vi "Evaluate Car Position.vi"(7 "Timeout":i32=-1, 11 "Car Wash Station Sequencer in":refnum<class "Car Wash Station Sequencer.lvclass">) -> (3 "Car Wash Station Sequencer out":refnum<class "Car Wash Station Sequencer.lvclass">, 5 "Timeout out":i32)   [LabVIEW 2016, in "CLD Exam - Car Wash.lvlib" / "Car Wash Station Sequencer.lvclass"]
uses:
  Car Wash Station Sequencer.lvclass
  D:/Repos/Stream/software/Mediator/Classes/Mediated Actor/Mediated Actor.lvclass
  Car Wash Station Sequencer.lvclass/Car Wash Station Sequencer.ctl
  Car Wash Finished Event/Car Wash Finished.lvclass
  D:/Repos/Stream/software/Mediator/Classes/Message Interface/Message Interface.lvclass
  Car Out of Position Event/Car Out of Position.lvclass
  Mediator/Classes/Message Interface/Message Interface.lvclass
  Car Wash Option Started Event/Car Wash Option Started.lvclass
  Mediator/Classes/Message Transport Queue/Message Transport Queue.lvclass
  Mediator/Classes/Mediated Actor/Mediated Actor.lvclass
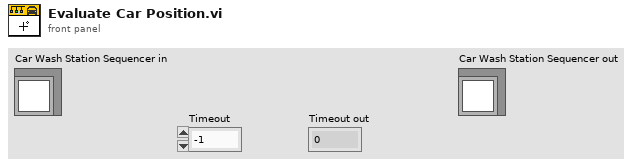
[diagram p1: front panel]
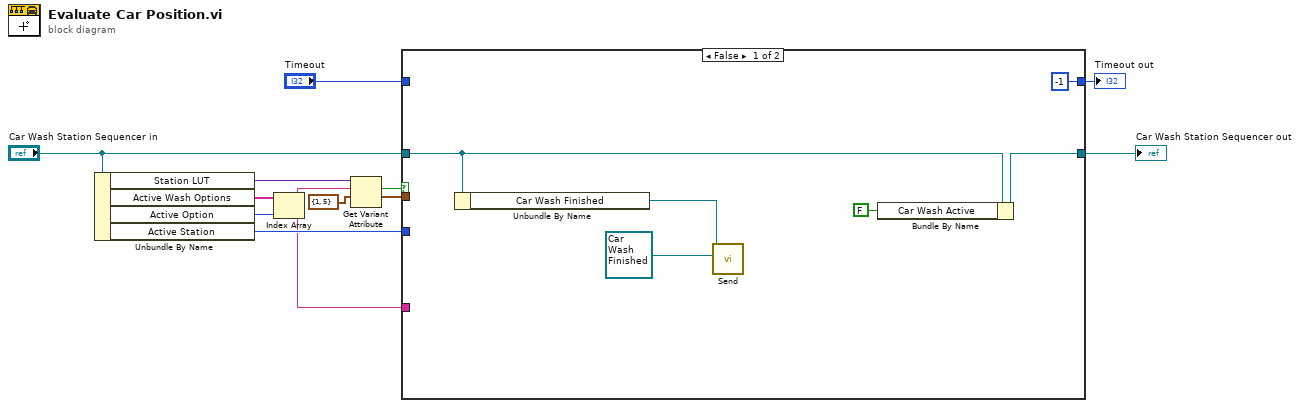
[diagram p0: block diagram]
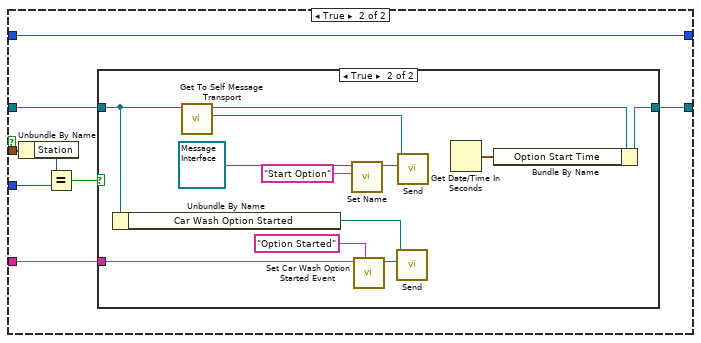
[diagram p2: hidden frame]
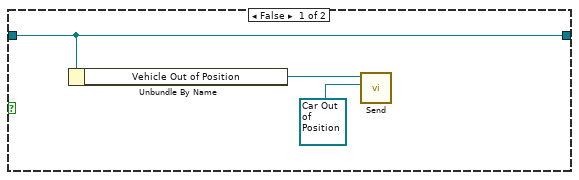
[diagram p3: hidden frame]
diagram:
  n1 = Unbundle By Name("Car Wash Station Sequencer in") -> ("Station LUT"=w10:variant, "Active Wash Options"=w12:string[], "Active Option"=w11:u8, "Active Station"=w7:u8)
  n2 = Index Array(array=w12, index=w11) -> (element=w4:string)
  n3 = Get Variant Attribute(Variant=w10, name=w4, default value (empty Variant)=cluster{"Station":u8, "Step Time":u16} {"Station"=1, "Step Time"=5}) -> (found=w3:bool, value=w8:cluster{"Station":u8, "Step Time":u16})  [unwired: 1 in, 2 out]
  n4 = case shown="False" w3 {
    tunnel: w8 -> [_ w26]
    tunnel: w7 -> [_ w24]
    tunnel: "Car Wash Station Sequencer in" -> [w15 w23]
    tunnel: [w14 w21] -> w5
    tunnel: w4 -> [_ w20]
    tunnel: [-1 ("Timeout") w19] -> w1
    tunnel: "Timeout" -> [_ w19]
    frame False {
      n5 = Unbundle By Name(w15) -> ("Car Wash Finished"=w18:refnum<class "Message Transport Queue.lvclass">)
      n6 = call-dynamic "Send.vi"("Message"=refnum<class "Car Wash Finished.lvclass"> refnum ("Car Wash Finished.lvclass"), "Message Transport Queue in"=w18) -> ()  [unwired: 7 in, 3 out]
      n7 = Bundle By Name(cluster=w15, "Car Wash Active"=FALSE ("Data.Car Wash Active")) -> (w14:refnum<class "Car Wash Station Sequencer.lvclass">)
    }
    frame True {
      n8 = Unbundle By Name(w26) -> ("Station"=w25:u8)
      n9 = Equal?(x=w25, y=w24) -> (x = y?=w22:bool)
      n10 = case shown="True" w22 {
        tunnel: w23 -> [w27 w37]
        tunnel: [w27 w31] -> w21
        tunnel: w20 -> [_ w36]
        frame False {
          n11 = Unbundle By Name(w27) -> ("Vehicle Out of Position"=w29:refnum<class "Message Transport Queue.lvclass">)
          n12 = call-dynamic "Send.vi"("Message"=refnum<class "Car Out of Position.lvclass"> refnum ("Car Out of Position.lvclass"), "Message Transport Queue in"=w29) -> ()  [unwired: 7 in, 3 out]
        }
        frame True {
          n13 = Unbundle By Name(w37) -> ("Car Wash Option Started"=w35:refnum<class "Message Transport Queue.lvclass">)
          n14 = call "Get To Self Message Transport.vi"("Mediated Actor in"=w37) -> ("To Self"=w41:refnum<class "Message Transport Queue.lvclass">, "Mediated Actor out"=w32:refnum<class "Car Wash Station Sequencer.lvclass">)  [unwired: 9 in]
          n15 = call "Set Name.vi"("Name"="Start Option", "Message Interface in"=refnum<class "Message Interface.lvclass"> refnum) -> ("Message Interface out"=w40:refnum<class "Message Interface.lvclass">)  [unwired: 8 in, 1 out]
          n16 = call "Set Car Wash Option Started Event.vi"("Name"="Option Started", "Option"=w36) -> ("Car Wash Option Started out"=w34:refnum<class "Car Wash Option Started.lvclass">)  [unwired: 9 in]
          n17 = call-dynamic "Send.vi"("Message"=w34, "Message Transport Queue in"=w35) -> ()  [unwired: 7 in, 3 out]
          n18 = call-dynamic "Send.vi"("Message"=w40, "Message Transport Queue in"=w41) -> ()  [unwired: 7 in, 3 out]
          n19 = Get Date/Time In Seconds() -> (seconds since 1Jan1904=w30:timestamp)
          n20 = Bundle By Name(cluster=w32, "Option Start Time"=w30) -> (w31:refnum<class "Car Wash Station Sequencer.lvclass">)
        }
      }
    }
  }
  "Car Wash Station Sequencer out" <- w5
  "Timeout out" <- w1
